vi "NoiseOutput_Host.vi"() -> ()   [LabVIEW 2012]
uses:
  <vilib>/DAQmx/write.llb/DAQmx Write (Analog 1D Wfm NChan NSamp).vi
  <vilib>/DAQmx/create/channels.llb/DAQmx Create Channel (AO-Voltage-Basic).vi
  <vilib>/DAQmx/configure/timing.llb/DAQmx Timing (Sample Clock).vi
  <vilib>/FPGAPlugInAG/PXI-7813R/niLvFpga_Open_PXI-7813R.vi
  <vilib>/rvi/interface/common/dynamic/niFpgaDynamicAddResources.vi
  <vilib>/DAQmx/miscellaneous.llb/DAQmx Fill In Error Info.vi
  <vilib>/Utility/error.llb/Error Cluster From Error Code.vi
  <vilib>/rvi/errors/niLvFpgaAdjustHostInterfaceError.vi
  <vilib>/FPGAPlugInAG/Dynamic/niLvFpga_Close_Dynamic.vi
  <vilib>/rvi/interface/nirviOpenFPGA/nirviOpenFPGA.xnode
  FPGA Bitfiles/NoiseOutput_FPGATarget_NoiseOutput_F7EC4DC8.lvbitx
  NoiseOutput.vi
  <vilib>/rvi/interface/nirviReadWriteControl/nirviReadWriteControl.xnode
  <vilib>/rvi/interface/nirviCloseFPGA/nirviCloseFPGA.xnode
  <vilib>/measure/NI_MABase.lvlib
  <vilib>/rvi/interface/Simulation/niFpgaSimulationCallBeginRW.vi
  NiFpgaLv.dll
panel:
  in  "Program trigger":bool
  in  "Stop":bool
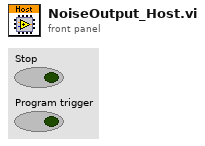
[diagram p1: front panel]
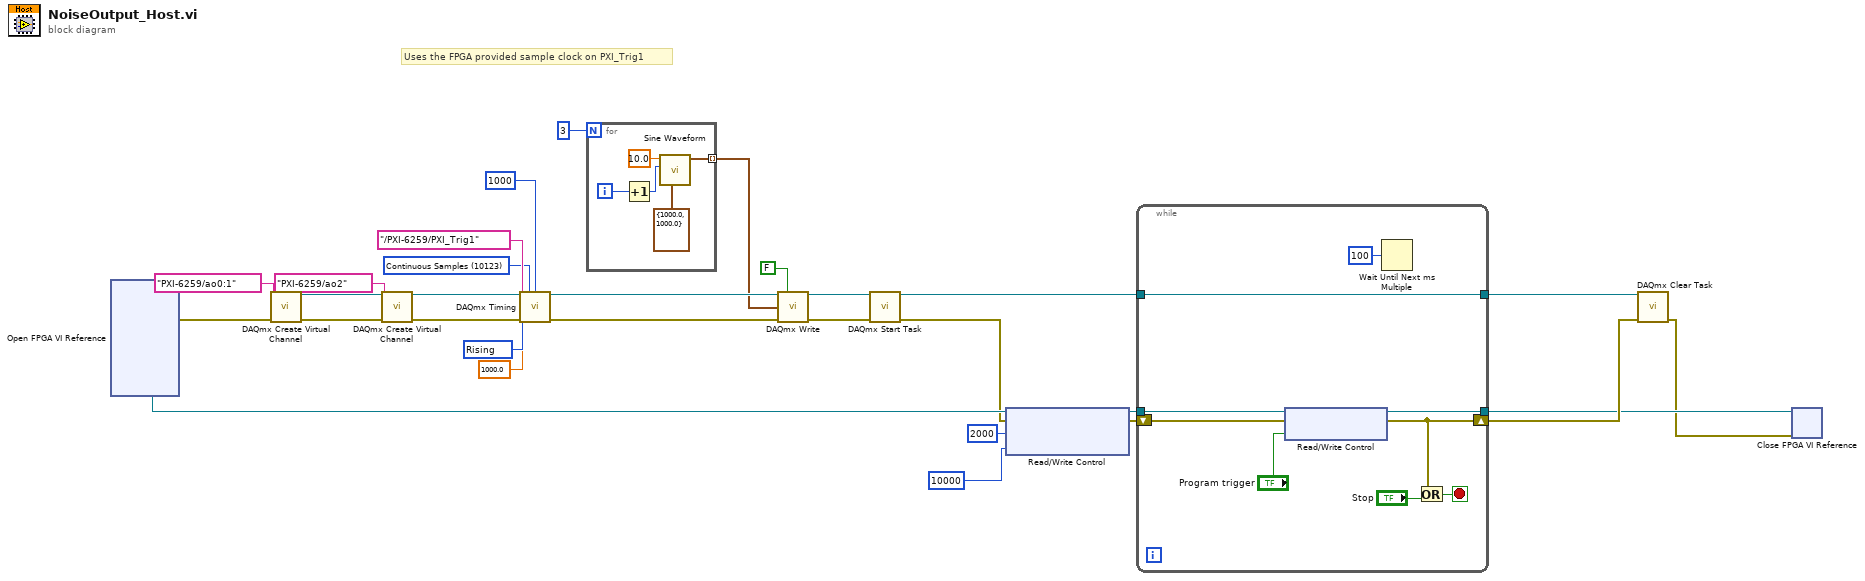
[diagram p0: block diagram]
diagram:
  w26 = 10123 items=["Finite Samples"=10178, "Continuous Samples"=10123, "Hardware Timed Single Point"=12522] ("sample mode")
  w28 = 10280 items=["Rising"=10280, "Falling"=10171] ("active edge")
  # "Uses the FPGA provided sample clock on PXI_Trig1"
  n1 = xnode "Open FPGA VI Reference"() -> ("FPGA VI Reference Out"=w8:refnum<k20>, "error out"=w12:errorcluster)  [unwired: 2 in]
  n2 = call-poly <vilib>:"DAQmx Create Virtual Channel.vi"("physical channels"=tag "PXI-6259/ao0:1", "error in"=w12) -> ("task out"=w18:refnum<k21>, "error out"=w15:errorcluster)  [unwired: 12 in]
  n3 = call-poly <vilib>:"DAQmx Create Virtual Channel.vi"("task in"=w18, "physical channels"=tag "PXI-6259/ao2", "error in"=w15) -> ("task out"=w17:refnum<k21>, "error out"=w16:errorcluster)  [unwired: 11 in]
  n4 = call-poly <vilib>:"DAQmx Timing.vi"("task/channels in"=w17, "sample mode"=w26, "samples per channel"=1000, "rate"=1000.0, "source"=tag "/PXI-6259/PXI_Trig1", "active edge"=w28, "error in"=w16) -> ("task out"=w24:refnum<k21>, "error out"=w25:errorcluster)  [unwired: 7 in]
  n5 = for {
    N: 3 -> [_]
    tunnel: [w33] -> w21 mode=indexing
    i -> [w32]
    n6 = Increment(x=w32) -> (x+1=w31:i32)
    n7 = call <vilib>:"Sine Waveform.vi"("sampling info"=cluster{"Fs":dbl, "#s":dbl} {"Fs"=1000.0, "#s"=1000.0}, "amplitude"=w31, "frequency"=10.0) -> ("signal out"=w33:waveform(dbl))  [unwired: 7 in, 1 out]
  }
  n8 = call-poly <vilib>:"DAQmx Write.vi"("task/channels in"=w24, "auto start"=FALSE, "data"=w21, "error in"=w25) -> ("task out"=w19:refnum<k21>, "error out"=w13:errorcluster)  [unwired: 9 in, 1 out]
  n9 = call <vilib>:"DAQmx Start Task.vi"("task/channels in"=w19, "error in"=w13) -> ("task out"=w11:refnum<k21>, "error out"=w4:errorcluster)  [unwired: 12 in]
  n10 = xnode "Read/Write Control"("FPGA VI Reference In"=w8, "error in"=w4, "Sample clock cycles"=u64 2000 ("Half clock cycles"), "Max sample pulses"=u64 10000) -> ("FPGA VI Reference Out"=w6:refnum<k20>, "error out"=w5:errorcluster)
  n11 = while {
    shift-right: [w38] -> w10
    shift-left: w5 -> [w39]
    tunnel: w11 -> [w44]
    tunnel: [w44] -> w9
    tunnel: w6 -> [w37]
    tunnel: [w36] -> w3
    stop <- w43 stop-if-true
    n12 = xnode "Read/Write Control"("FPGA VI Reference In"=w37, "error in"=w39, "Program trigger"="Program trigger") -> ("FPGA VI Reference Out"=w36:refnum<k20>, "error out"=w38:errorcluster)
    n13 = Wait Until Next ms Multiple(millisecond multiple=u32 100) -> ()  [unwired: 1 out]
    n14 = Or(x=w38, y="Stop") -> (x .or. y?=w43:bool)
  }
  n15 = call <vilib>:"DAQmx Clear Task.vi"("task in"=w9, "error in"=w10) -> ("error out"=w2:errorcluster)  [unwired: 13 in]
  n16 = xnode "Close FPGA VI Reference"("FPGA VI Reference In"=w3, "error in"=w2) -> ()  [unwired: 1 out]
